vi "Notstop VI.vi"(8 "error in":errorcluster) -> (0 "error out":errorcluster)   [LabVIEW 2016]
uses:
  Globale Variablen VI/AutonomousMode.vi
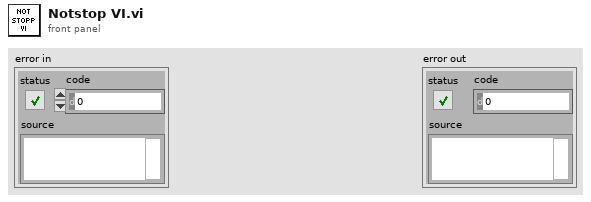
[diagram p1: front panel]
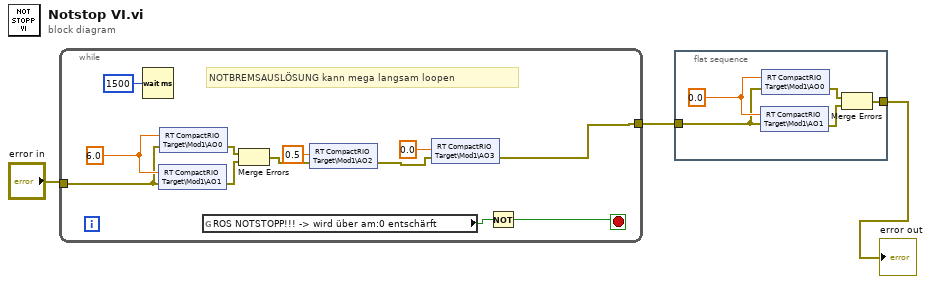
[diagram p0: block diagram]
diagram:
  n1 = while {
    tunnel: [w4] -> w2
    tunnel: "error in" -> [w5]
    stop <- w6 stop-if-true
    w14 = 6.0
    # "NOTBREMSAUSLÖSUNG kann mega langsam loopen"
    n2 = Wait (ms)(milliseconds to wait=u32 1500) -> ()  [unwired: 1 out]
    n3 = shared-variable "RT CompactRIO Target\\Mod1\\AO1"(w14, error in=w5) -> (error out=w13:errorcluster)
    n4 = shared-variable "RT CompactRIO Target\\Mod1\\AO0"(w14, error in=w5) -> (error out=w12:errorcluster)
    n5 = global read "AutonomousMode.vi" "ROS NOTSTOPP!!! -> wird über am:0 entschärft"() -> (w7:bool)
    n6 = Merge Errors(w12, w13) -> (w11:errorcluster)
    n7 = shared-variable "RT CompactRIO Target\\Mod1\\AO2"(0.5, error in=w11) -> (error out=w9:errorcluster)
    n8 = shared-variable "RT CompactRIO Target\\Mod1\\AO3"(0.0, error in=w9) -> (error out=w4:errorcluster)
    n9 = Not(x=w7) -> (.not. x?=w6:bool)
  }
  n10 = flat-sequence {
    tunnel: w2 -> [w19]
    tunnel: [w16] -> w1
    frame #0 {
      w20 = 0.0
      n11 = shared-variable "RT CompactRIO Target\\Mod1\\AO1"(w20, error in=w19) -> (error out=w17:errorcluster)
      n12 = shared-variable "RT CompactRIO Target\\Mod1\\AO0"(w20, error in=w19) -> (error out=w18:errorcluster)
      n13 = Merge Errors(w18, w17) -> (w16:errorcluster)
    }
  }
  "error out" <- w1
